vi "Write Analogue.vi"(8 "error in (no error)":errorcluster, 9 "output":bool, 10 "Channel index":i32, 11 "PS Instrument":refnum<class "Power Supply Instrument.lvclass">) -> (0 "error out":errorcluster, 2 "Success?":bool=TRUE, 3 "PS Instrument out":refnum<class "Power Supply Instrument.lvclass">)   [LabVIEW 2025, in "Power Supply.lvlib" / "Power Supply Instrument.lvclass"]
uses:
  Power Supply Instrument.lvclass
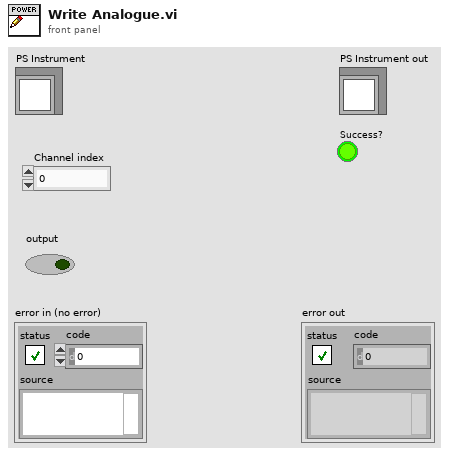
[diagram p1: front panel]
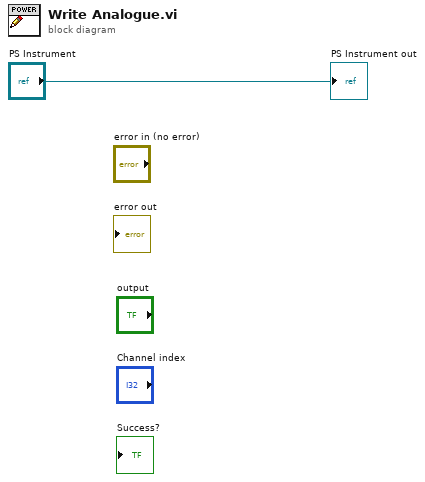
[diagram p0: block diagram]
diagram:
  "PS Instrument out" <- "PS Instrument"
